vi "Parse.vi"(8 "error in (no error)":errorcluster, 11 "PathCommands.MoveTo in":refnum<class "PathCommands.MoveTo.lvclass">) -> (0 "error out":errorcluster, 3 "PathCommands.MoveTo out":refnum<class "PathCommands.MoveTo.lvclass">)   [LabVIEW 2019, in "PathCommands.MoveTo.lvclass"]
uses:
  PathCommands.MoveTo.lvclass
  PathCommands/Point.ctl
  <vilib>/Utility/error.llb/whitespace.ctl
  PathCommands/PathCommands.lvclass
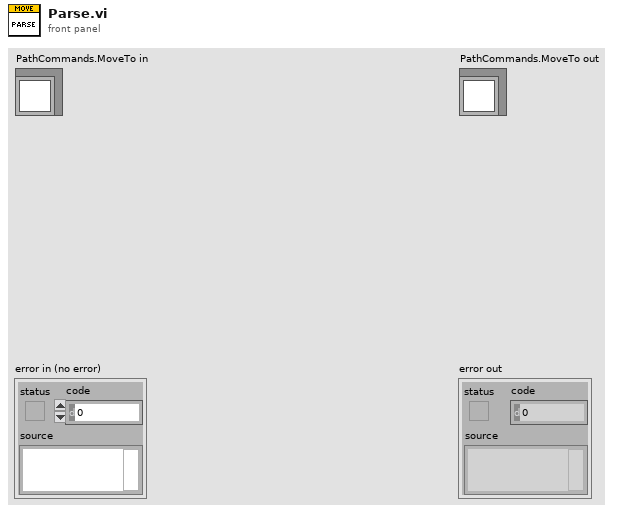
[diagram p1: front panel]
types:
  T1 = typedef "whitespace.ctl" = u16
  T2 = typedef "PathCommands.lvclass/Point.ctl" = cluster{"X":dbl, "Y":dbl}
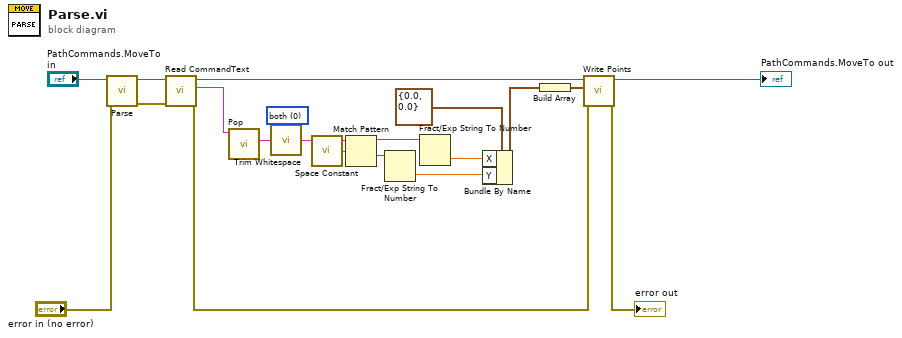
[diagram p0: block diagram]
diagram:
  w2 = T1 0 items=["both", "start of string", "end of string"] ("location (both)")
  n1 = call-parent "Parse.vi"("error in (no error)"="error in (no error)", "PathCommands in"="PathCommands.MoveTo in") -> ("error out"=w5:errorcluster, "PathCommands out"=w18:refnum<class "PathCommands.MoveTo.lvclass">)  [unwired: 8 in]
  n2 = call-dynamic "Read CommandText.vi"("error in (no error)"=w5, "PathCommands in"=w18) -> ("error out"=w4:errorcluster, "CommandText"=w17:string, "PathCommands out"=w10:refnum<class "PathCommands.MoveTo.lvclass">)  [unwired: 7 in]
  n3 = call "Pop.vi"("Command Text"=w17) -> ("Command Info"=w16:string)  [unwired: 9 in, 1 out]
  n4 = call <vilib>:"Trim Whitespace.vi"("string"=w16, "location (both)"=w2) -> ("trimmed string"=w3:string)
  n5 = call <vilib>:"Space Constant.vi"() -> ("String"=w1:string)
  n6 = Match Pattern(string=w3, regular expression=w1) -> (before substring=w15:string, after substring=w14:string)  [unwired: 1 in, 2 out]
  n7 = Fract/Exp String To Number(string=w14) -> (number=w11:dbl)  [unwired: 3 in, 1 out]
  n8 = Fract/Exp String To Number(string=w15) -> (number=w12:dbl)  [unwired: 3 in, 1 out]
  n9 = Bundle By Name(cluster=T2 {"X"=0.0, "Y"=0.0} ("Point"), "X"=w12, "Y"=w11) -> (w7:T2)
  n10 = Build Array(w7) -> (w8:T2[])
  n11 = call-dynamic "Write Points.vi"("error in (no error)"=w4, "Points"=w8, "PathCommands in"=w10) -> ("error out"=→"error out":errorcluster, "PathCommands out"=→"PathCommands.MoveTo out":refnum<class "PathCommands.MoveTo.lvclass">)  [unwired: 7 in]
